vi "BCU诊断标定.vi"(8 "CAN端口":u16(ring), 9 "设备索引号":u16(ring), 10 "CAN卡类型":u32(ring)=21) -> ()   [LabVIEW 2013] (continued)
                  n4261 = call "多帧发送机制(EV05).vi"("can卡类型"=w6108, "设备索引号"=w6107, "CAN端口"=w6106, "命令"=w6105, "板号"=w6102, "命令序号"=w6104, "输入数据"=dbl[] [0.0]) -> ()  [unwired: 1 in, 12 out]
                  n4262 = local write "命令序号"(w6104) -> ()
                }
              }
            }
            frame #1 {
              n4263 = while {
                tunnel: [w6110] -> w6109
                i -> [w6115]
                stop <- w6112 stop-if-true
                n4264 = global read "EV05全局变量1.vi" "写入超时"() -> (w6110:bool)
                n4265 = Greater Or Equal?(x=w6115, y=25) -> (x >= y?=w6113:bool)
                n4266 = Or(x=w6110, y=w6113) -> (x .or. y?=w6112:bool)
                n4267 = Wait Until Next ms Multiple(millisecond multiple=u32 100 ("毫秒倍数")) -> ()  [unwired: 1 out]
              }
            }
            frame #2 {
              n4268 = case shown="假" w6116 {
                frame False {
                  n4269 = control-ref of="结果"() -> (w6118:refnum<vi>)
                  n4270 = Concatenate Strings("项目软件版本" ("字符串"), "     读取失败" ("字符串")) -> (w6121:string)
                  n4271 = Build Array(w6121) -> (w6120:string[])
                  n4272 = call "表格编辑(版本读取).vi"("新元素/子数组"=w6120, "活动单元格:单元格背景色"=u32 16740749, "MCListbox引用句柄"=w6118) -> ()  [unwired: 9 out]
                }
                frame True {
                }
              }
              n4273 = call <vilib>:"Unset Busy.vi"() -> ()  [unwired: 2 in, 10 out]
            }
          }
        }
        frame "读取故障状态" {
          n4274 = stacked-sequence {
            seq-local: [_ w6147 _] -> [_ _ w6154]
            frame #0 {
              n4275 = local read "设备索引号"() -> (w6124:u16)
              n4276 = local read "CAN卡类型"() -> (w6125:u32)
              n4277 = local read "CAN端口"() -> (w6123:u16)
              n4278 = stacked-sequence {
                tunnel: w6125 -> [w6128 w6137]
                tunnel: w6124 -> [w6127 w6136]
                tunnel: w6123 -> [w6126 w6135]
                frame #0 {
                  n4279 = dll-call lib="PTH1mabs FBluewave New EnergySVN_WorkBMS_Monitor_Bnet01trunk参数设置data\nkerneldlls\nusbcan.dll" fn="VCI_ClearBuffer"("DeviceType"=w6128, "DeviceInd"=w6127, "CANInd"=w6126) -> (error out=w6129:errorcluster)  [unwired: 4 in, 4 out]
                  n4280 = call <vilib>:"Clear Errors.vi"("error in (no error)"=w6129) -> ()  [unwired: 6 in, 1 out]
                }
                frame #1 {
                  n4281 = local read "从板板号 2"() -> (w6130:u8)
                  n4282 = case shown="1..30" w6130 {
                    tunnel: [u8 133 ("命令") u8 4 ("命令")] -> w6134
                    frame 0, Default {
                    }
                    frame 1..30 {
                    }
                  }
                  n4283 = local read "状态选择"() -> (w6132:T18)
                  n4284 = local write "命令"(w6134) -> ()
                  n4285 = case shown="\"预充电故障,继电器驱动故障\"" w6132 {
                    tunnel: [1 2 3 4 5 6 7] -> w6131
                    frame "电压,内总电压,外总电压,温度,电流,绝缘,系统时钟,充电均衡,放电均衡", Default {
                    }
                    frame "CPU,CPU内部EE存储器,CPU内部FLASH,内部EE存储器,45db存储器" {
                    }
                    frame "CAN检测故障" {
                    }
                    frame "软件故障" {
                    }
                    frame "RS485,RS232检测故障" {
                    }
                    frame "DI,DO,AI,AO检测故障" {
                    }
                    frame "预充电故障,继电器驱动故障" {
                    }
                  }
                  n4286 = call "多帧发送机制(EV05).vi"("can卡类型"=w6137, "设备索引号"=w6136, "CAN端口"=w6135, "命令"=w6134, "板号"=w6130, "命令序号"=w6131, "输入数据"=dbl[] [0.0]) -> ()  [unwired: 1 in, 12 out]
                  n4287 = local write "命令序号"(w6131) -> ()
                }
              }
            }
            frame #1 {
              n4288 = while {
                tunnel: [w6148] -> w6147
                i -> [w6153]
                stop <- w6150 stop-if-true
                n4289 = global read "EV05全局变量1.vi" "写入超时"() -> (w6148:bool)
                n4290 = Greater Or Equal?(x=w6153, y=25) -> (x >= y?=w6151:bool)
                n4291 = Or(x=w6148, y=w6151) -> (x .or. y?=w6150:bool)
                n4292 = Wait Until Next ms Multiple(millisecond multiple=u32 100 ("毫秒倍数")) -> ()  [unwired: 1 out]
              }
            }
            frame #2 {
              n4293 = case shown="真" w6154 {
                frame False {
                  n4294 = Concatenate Strings("故障信息" ("字符串"), "     读取失败" ("字符串")) -> (w6156:string)
                  n4295 = One Button Dialog(message=w6156, button name ("OK")="确定" ("按钮名称（“确定”）")) -> ()  [unwired: 1 out]
                }
                frame True {
                  n4296 = One Button Dialog(message="故障信息读取完成" ("字符串"), button name ("OK")="确定" ("按钮名称（“确定”）")) -> ()  [unwired: 1 out]
                }
              }
              n4297 = call <vilib>:"Unset Busy.vi"() -> ()  [unwired: 2 in, 10 out]
            }
          }
        }
        frame "平台软件版本读取" {
          n4298 = stacked-sequence {
            seq-local: [_ w6176 _] -> [_ _ w6183]
            frame #0 {
              n4299 = local read "设备索引号"() -> (w6163:u16)
              n4300 = local read "CAN卡类型"() -> (w6164:u32)
              n4301 = local read "CAN端口"() -> (w6162:u16)
              n4302 = stacked-sequence {
                tunnel: w6164 -> [w6167 w6175]
                tunnel: w6163 -> [w6166 w6174]
                tunnel: w6162 -> [w6165 w6173]
                tunnel: u8 137 ("命令") -> [_ w6172]
                frame #0 {
                  n4303 = dll-call lib="PTH1mabs FBluewave New EnergySVN_WorkBMS_Monitor_Bnet01trunk参数设置data\nkerneldlls\nusbcan.dll" fn="VCI_ClearBuffer"("DeviceType"=w6167, "DeviceInd"=w6166, "CANInd"=w6165) -> (error out=w6168:errorcluster)  [unwired: 4 in, 4 out]
                  n4304 = call <vilib>:"Clear Errors.vi"("error in (no error)"=w6168) -> ()  [unwired: 6 in, 1 out]
                }
                frame #1 {
                  w6171 = u32 2 ("命令序号")
                  n4305 = local read "从板板号"() -> (w6169:u8)
                  n4306 = local write "命令"(w6172) -> ()
                  n4307 = call "多帧发送机制(EV05).vi"("can卡类型"=w6175, "设备索引号"=w6174, "CAN端口"=w6173, "命令"=w6172, "板号"=w6169, "命令序号"=w6171, "输入数据"=dbl[] [0.0]) -> ()  [unwired: 1 in, 12 out]
                  n4308 = local write "命令序号"(w6171) -> ()
                }
              }
            }
            frame #1 {
              n4309 = while {
                tunnel: [w6177] -> w6176
                i -> [w6182]
                stop <- w6179 stop-if-true
                n4310 = global read "EV05全局变量1.vi" "写入超时"() -> (w6177:bool)
                n4311 = Greater Or Equal?(x=w6182, y=25) -> (x >= y?=w6180:bool)
                n4312 = Or(x=w6177, y=w6180) -> (x .or. y?=w6179:bool)
                n4313 = Wait Until Next ms Multiple(millisecond multiple=u32 100 ("毫秒倍数")) -> ()  [unwired: 1 out]
              }
            }
            frame #2 {
              n4314 = case shown="假" w6183 {
                frame False {
                  n4315 = control-ref of="结果"() -> (w6186:refnum<vi>)
                  n4316 = Concatenate Strings("平台软件版本" ("字符串"), "     读取失败" ("字符串")) -> (w6188:string)
                  n4317 = Build Array(w6188) -> (w6185:string[])
                  n4318 = call "表格编辑(版本读取).vi"("新元素/子数组"=w6185, "活动单元格:单元格背景色"=u32 16740749, "MCListbox引用句柄"=w6186) -> ()  [unwired: 9 out]
                }
                frame True {
                }
              }
              n4319 = call <vilib>:"Unset Busy.vi"() -> ()  [unwired: 2 in, 10 out]
            }
          }
        }
        frame "模块软件版本读取" {
          n4320 = local read "从板板号"() -> (w6190:u8)
          n4321 = local read "模块软件版本"() -> (w6191:T1)
          n4322 = case shown="\"全部读取\"" w6191 {
            selector: w6191 -> [w6192 w6236]
            tunnel: w6190 -> [_ w6235]
            frame "BCUMCAL", Default {
              n4323 = stacked-sequence {
                seq-local: [_ _ w6218 _] -> [_ _ _ w6225]
                tunnel: w6192 -> [_ w6198 _ w6226]
                frame #0 {
                  w6197 = FALSE ("写?")
                  n4324 = call <vilib>:"Set Busy.vi"("disable click? (T)"=FALSE) -> ()  [unwired: 3 in, 8 out]
                  n4325 = local write "写?"(w6197) -> ()
                  n4326 = global write "EV05全局变量1.vi" "流控帧 2"(TRUE ("流控帧 2")) -> ()
                  n4327 = global write "EV05全局变量1.vi" "写入超时"(w6197) -> ()
                  n4328 = local write "控制1"(TRUE ("控制1")) -> ()
                  n4329 = local write "消除"(TRUE ("消除")) -> ()
                }
                frame #1 {
                  n4330 = Quotient & Remainder(x=w6198, y=256) -> (x-y*floor(x/y)=w6199:i32, floor(x/y)=w6200:i32)
                  n4331 = Build Array(w6200, w6199, u8 0 ("板号")) -> (w6203:i32[])
                  n4332 = local read "设备索引号"() -> (w6205:u16)
                  n4333 = local read "CAN卡类型"() -> (w6206:u32)
                  n4334 = local read "CAN端口"() -> (w6204:u16)
                  n4335 = stacked-sequence {
                    tunnel: w6206 -> [w6209 w6217]
                    tunnel: w6205 -> [w6208 w6216]
                    tunnel: w6204 -> [w6207 w6215]
                    tunnel: w6203 -> [_ w6214]
                    frame #0 {
                      n4336 = dll-call lib="PTH1mabs FBluewave New EnergySVN_WorkBMS_Monitor_Bnet01trunk参数设置data\nkerneldlls\nusbcan.dll" fn="VCI_ClearBuffer"("DeviceType"=w6209, "DeviceInd"=w6208, "CANInd"=w6207) -> (error out=w6210:errorcluster)  [unwired: 4 in, 4 out]
                      n4337 = call <vilib>:"Clear Errors.vi"("error in (no error)"=w6210) -> ()  [unwired: 6 in, 1 out]
                    }
                    frame #1 {
                      w6213 = u8 137 ("命令")
                      w6211 = u32 3 ("命令序号")
                      n4338 = local read "从板板号"() -> (w6212:u8)
                      n4339 = local write "命令"(w6213) -> ()
                      n4340 = call "多帧发送机制(EV05).vi"("can卡类型"=w6217, "设备索引号"=w6216, "CAN端口"=w6215, "命令"=w6213, "板号"=w6212, "命令序号"=w6211, "输入数据"=w6214) -> ()  [unwired: 1 in, 12 out]
                      n4341 = local write "命令序号"(w6211) -> ()
                    }
                  }
                }
                frame #2 {
                  n4342 = while {
                    tunnel: [w6219] -> w6218
                    i -> [w6224]
                    stop <- w6220 stop-if-true
                    n4343 = global read "EV05全局变量1.vi" "写入超时"() -> (w6219:bool)
                    n4344 = Greater Or Equal?(x=w6224, y=25) -> (x >= y?=w6221:bool)
                    n4345 = Or(x=w6219, y=w6221) -> (x .or. y?=w6220:bool)
                    n4346 = Wait Until Next ms Multiple(millisecond multiple=u32 100 ("毫秒倍数")) -> ()  [unwired: 1 out]
                  }
                }
                frame #3 {
                  n4347 = call <vilib>:"Unset Busy.vi"() -> ()  [unwired: 2 in, 10 out]
                  n4348 = case shown="假" w6225 {
                    tunnel: w6226 -> [w6228 _]
                    frame False {
                      n4349 = Number To Decimal String(number=w6228) -> (decimal integer string=w6229:string)  [unwired: 1 out]
                      n4350 = control-ref of="结果"() -> (w6230:refnum<vi>)
                      n4351 = Concatenate Strings("模块" ("字符串"), w6229, "     读取失败" ("字符串")) -> (w6233:string)
                      n4352 = Build Array(w6233) -> (w6232:string[])
                      n4353 = call "表格编辑(版本读取).vi"("新元素/子数组"=w6232, "活动单元格:单元格背景色"=u32 16740749, "MCListbox引用句柄"=w6230) -> ()  [unwired: 9 out]
                    }
                    frame True {
                    }
                  }
                }
              }
            }
            frame "全部读取" {
              n4354 = stacked-sequence {
                seq-local: [w6237 _] -> [_ w6275]
                tunnel: w6236 -> [_ w6277]
                tunnel: w6235 -> [w6238 w6276]
                frame #0 {
                  n4355 = stacked-sequence {
                    tunnel: w6238 -> [_ w6247 _]
                    tunnel: [_ _ w6267] -> w6237
                    frame #0 {
                      w6243 = FALSE ("写?")
                      n4356 = control-ref of="模块软件版本 2"() -> (w6241:refnum<vi>)
                      n4357 = call <vilib>:"Set Busy.vi"("disable click? (T)"=FALSE) -> ()  [unwired: 3 in, 8 out]
                      n4358 = local write "写?"(w6243) -> ()
                      n4359 = property class="MCListbox (严格)"(reference=w6241, "ItemNames"=string[][] []) -> ()  [unwired: 1 in, 2 out]
                      n4360 = global write "EV05全局变量1.vi" "写入超时"(w6243) -> ()
                      n4361 = local write "消除"(TRUE ("消除")) -> ()
                      n4362 = local write "控制1"(TRUE ("控制1")) -> ()
                      n4363 = global write "EV05全局变量1.vi" "流控帧 2"(TRUE ("流控帧 2")) -> ()
                      n4364 = local write "MODEL号"(u8[] [] ("MODEL号")) -> ()
                    }
                    frame #1 {
                      n4365 = local read "设备索引号"() -> (w6249:u16)
                      n4366 = local read "CAN卡类型"() -> (w6250:u32)
                      n4367 = local read "CAN端口"() -> (w6248:u16)
                      n4368 = stacked-sequence {
                        tunnel: w6250 -> [w6253 w6266]
                        tunnel: w6249 -> [w6252 w6265]
                        tunnel: w6248 -> [w6251 w6264]
                        tunnel: w6247 -> [_ w6256]
                        frame #0 {
                          n4369 = dll-call lib="PTH1mabs FBluewave New EnergySVN_WorkBMS_Monitor_Bnet01trunk参数设置data\nkerneldlls\nusbcan.dll" fn="VCI_ClearBuffer"("DeviceType"=w6253, "DeviceInd"=w6252, "CANInd"=w6251) -> (error out=w6254:errorcluster)  [unwired: 4 in, 4 out]
                          n4370 = call <vilib>:"Clear Errors.vi"("error in (no error)"=w6254) -> ()  [unwired: 6 in, 1 out]
                        }
                        frame #1 {
                          w6262 = u8 137 ("命令")
                          w6260 = u32 3 ("命令序号")
                          n4371 = Quotient & Remainder(x=u8 0 ("板号"), y=256) -> (x-y*floor(x/y)=w6257:i32, floor(x/y)=w6258:i32)
                          n4372 = local write "命令"(w6262) -> ()
                          n4373 = Build Array(w6258, w6257, u8 0 ("板号")) -> (w6263:i32[])
                          n4374 = call "多帧发送机制(EV05).vi"("can卡类型"=w6266, "设备索引号"=w6265, "CAN端口"=w6264, "命令"=w6262, "板号"=w6256, "命令序号"=w6260, "输入数据"=w6263) -> ()  [unwired: 1 in, 12 out]
                          n4375 = local write "命令序号"(w6260) -> ()
                        }
                      }
                    }
                    frame #2 {
                      n4376 = while {
                        tunnel: [w6269] -> w6267
                        i -> [w6273]
                        stop <- w6270 stop-if-true
                        n4377 = local read "强制停止版本读取"() -> (w6268:bool)
                        n4378 = global read "EV05全局变量1.vi" "写入超时"() -> (w6269:bool)
                        n4379 = Greater Or Equal?(x=w6273, y=35) -> (x >= y?=w6271:bool)
                        n4380 = Compound Arithmetic op=OR(w6268, w6269, w6271) -> (w6270:bool)
                        n4381 = Wait Until Next ms Multiple(millisecond multiple=u32 100 ("毫秒倍数")) -> ()  [unwired: 1 out]
                      }
                    }
                  }
                }
                frame #1 {
                  n4382 = case shown="真" w6275 {
                    tunnel: w6277 -> [_ w6287]
                    tunnel: w6276 -> [_ w6286]
                    frame False {
                      n4383 = control-ref of="结果"() -> (w6279:refnum<vi>)
                      n4384 = Concatenate Strings("模块编号" ("字符串"), "读取失败" ("字符串")) -> (w6282:string)
                      n4385 = Build Array(w6282) -> (w6281:string[])
                      n4386 = call "表格编辑(版本读取).vi"("新元素/子数组"=w6281, "活动单元格:单元格背景色"=u32 16740749, "MCListbox引用句柄"=w6279) -> ()  [unwired: 9 out]
                      n4387 = call <vilib>:"Unset Busy.vi"() -> ()  [unwired: 11 in, 1 out]
                    }
                    frame True {
                      n4388 = local read "MODEL号"() -> (w6285:u8[])
                      n4389 = Array Size(array=w6285) -> (size(s)=w6284:i32)
                      n4390 = for {
                        tunnel: w6287 -> [_]
                        tunnel: w6286 -> [w6290]
                        tunnel: w6285 -> [w6289] mode=indexing
                        tunnel: w6284 -> [w6288]
                        i -> [w6292]
                        n4391 = Increment(x=w6292) -> (x+1=w6291:i32)
                        n4392 = stacked-sequence {
                          seq-local: [_ _ _ w6319 _ _] -> [_ _ _ _ w6328 _]
                          seq-local: [_ w6298 _ _ _ _] -> [_ _ _ _ w6327 _]
                          tunnel: w6291 -> [_ _ _ _ _ w6339]
                          tunnel: w6289 -> [_ w6298 _ _ _ _]
                          tunnel: w6290 -> [_ w6299 _ _ _ _]
                          tunnel: w6288 -> [_ _ _ _ _ w6337]
                          frame #0 {
                            w6294 = FALSE ("写?")
                            n4393 = call <vilib>:"Set Busy.vi"("disable click? (T)"=FALSE) -> ()  [unwired: 3 in, 8 out]
                            n4394 = local write "写?"(w6294) -> ()
                            n4395 = global write "EV05全局变量1.vi" "写入超时"(w6294) -> ()
                            n4396 = global write "EV05全局变量1.vi" "流控帧 2"(TRUE ("流控帧 2")) -> ()
                            n4397 = local write "控制1"(TRUE ("控制1")) -> ()
                            n4398 = local write "消除"(TRUE ("消除")) -> ()
                          }
                          frame #1 {
                            n4399 = local read "设备索引号"() -> (w6301:u16)
                            n4400 = local read "CAN卡类型"() -> (w6302:u32)
                            n4401 = local read "CAN端口"() -> (w6300:u16)
                            n4402 = stacked-sequence {
                              tunnel: w6302 -> [w6305 w6318]
                              tunnel: w6301 -> [w6304 w6317]
                              tunnel: w6300 -> [w6303 w6316]
                              tunnel: w6299 -> [_ w6308]
                              tunnel: w6298 -> [_ w6307]
                              frame #0 {
                                n4403 = dll-call lib="PTH1mabs FBluewave New EnergySVN_WorkBMS_Monitor_Bnet01trunk参数设置data\nkerneldlls\nusbcan.dll" fn="VCI_ClearBuffer"("DeviceType"=w6305, "DeviceInd"=w6304, "CANInd"=w6303) -> (error out=w6306:errorcluster)  [unwired: 4 in, 4 out]
                                n4404 = call <vilib>:"Clear Errors.vi"("error in (no error)"=w6306) -> ()  [unwired: 6 in, 1 out]
                              }
                              frame #1 {
                                w6314 = u8 137 ("命令")
                                w6312 = u32 3 ("命令序号")
                                n4405 = Quotient & Remainder(x=w6307, y=256) -> (x-y*floor(x/y)=w6309:i32, floor(x/y)=w6310:i32)
                                n4406 = local write "命令"(w6314) -> ()
                                n4407 = Build Array(w6310, w6309, u8 0 ("板号")) -> (w6315:i32[])
                                n4408 = call "多帧发送机制(EV05).vi"("can卡类型"=w6318, "设备索引号"=w6317, "CAN端口"=w6316, "命令"=w6314, "板号"=w6308, "命令序号"=w6312, "输入数据"=w6315) -> ()  [unwired: 1 in, 12 out]
                                n4409 = local write "命令序号"(w6312) -> ()
                              }
                            }
                          }
                          frame #2 {
                          }
                          frame #3 {
                            n4410 = while {
                              tunnel: [w6321] -> w6319
                              i -> [w6325]
                              stop <- w6322 stop-if-true
                              n4411 = local read "强制停止版本读取"() -> (w6320:bool)
                              n4412 = global read "EV05全局变量1.vi" "写入超时"() -> (w6321:bool)
                              n4413 = Greater Or Equal?(x=w6325, y=25) -> (x >= y?=w6323:bool)
                              n4414 = Compound Arithmetic op=OR(w6320, w6321, w6323) -> (w6322:bool)
                              n4415 = Wait Until Next ms Multiple(millisecond multiple=u32 100 ("毫秒倍数")) -> ()  [unwired: 1 out]
                            }
                          }
                          frame #4 {
                            n4416 = call <vilib>:"Unset Busy.vi"() -> ()  [unwired: 11 in, 1 out]
                            n4417 = case shown="假" w6328 {
                              tunnel: w6327 -> [w6330 _]
                              frame False {
                                n4418 = control-ref of="结果"() -> (w6332:refnum<vi>)
                                n4419 = Number To Decimal String(number=w6330) -> (decimal integer string=w6331:string)  [unwired: 1 out]
                                n4420 = Concatenate Strings("模块" ("字符串"), w6331, "     读取失败" ("字符串")) -> (w6335:string)
                                n4421 = Build Array(w6335) -> (w6334:string[])
                                n4422 = call "表格编辑(版本读取).vi"("新元素/子数组"=w6334, "活动单元格:单元格背景色"=u32 16740749, "MCListbox引用句柄"=w6332) -> ()  [unwired: 9 out]
                              }
                              frame True {
                              }
                            }
                          }
                          frame #5 {
                            n4423 = Equal?(x=w6337, y=w6339) -> (x = y?=w6338:bool)
                            n4424 = case shown="真" w6338 {
                              frame False {
                              }
                              frame True {
                                n4425 = control-ref of="模块软件版本 2"() -> (w6350:refnum<vi>)
                                n4426 = local read "模块版本名称"() -> (w6349:string[][])
                                n4427 = local read "模块版本值"() -> (w6345:string[][])
                                n4428 = control-ref of="结果"() -> (w6357:refnum<vi>)
                                n4429 = property class="MCListbox (严格)"(reference=w6350) -> ("ItemNames"=w6353:string[][])  [unwired: 1 in, 2 out]
                                n4430 = local read "从板板号"() -> (w6340:u8)
                                n4431 = Concatenate Strings("模块版本读取完成" ("字符串")) -> (w6360:string)
                                n4432 = Build Array(w6360) -> (w6359:string[])
                                n4433 = call "表格编辑(版本读取).vi"("新元素/子数组"=w6359, "活动单元格:单元格背景色"=u32 21937, "MCListbox引用句柄"=w6357) -> ()  [unwired: 9 out]
                                n4434 = Transpose 2D Array(2D array=w6353) -> (transposed array=w6354:string[][])
                                n4435 = local write "强制停止版本读取"(FALSE ("强制停止 2")) -> ()
                                n4436 = local read "模块个数"() -> (w6343:u8[])
                                n4437 = Index Array(array=w6354, index (row) #1=0 ("索引 (行)"), index (row) #2=1 ("索引 (行)")) -> (element #1=w6344:string[], element #2=w6346:string[])  [unwired: 2 in]
                                n4438 = Replace Array Subset(array=w6349, new element=w6344, index (row)=w6340) -> (w6348:string[][])  [unwired: 1 in]
                                n4439 = Replace Array Subset(array=w6345, new element=w6346, index (row)=w6340) -> (w6347:string[][])  [unwired: 1 in]
                                n4440 = local write "模块版本名称"(w6348) -> ()
                                n4441 = local write "模块版本值"(w6347) -> ()
                                n4442 = Array Size(array=w6344) -> (size(s)=w6341:i32)
                                n4443 = Replace Array Subset(array=w6343, new element=w6341, index=w6340) -> (w6342:u8[])
                                n4444 = local write "模块个数"(w6342) -> ()
                              }
                            }
                          }
                        }
                      }
                    }
                  }
                }
              }
            }
          }
        }
        frame "硬件版本读取" {
          n4445 = stacked-sequence {
            seq-local: [_ _ w6368 _] -> [_ _ _ w6375]
            frame #0 {
              w6364 = u8 137 ("命令")
              w6363 = u32 4 ("命令序号")
              n4446 = local read "设备索引号"() -> (w6366:u16)
              n4447 = local read "CAN卡类型"() -> (w6367:u32)
              n4448 = local read "CAN端口"() -> (w6365:u16)
              n4449 = local read "从板板号"() -> (w6361:u8)
              n4450 = local write "命令"(w6364) -> ()
              n4451 = call "多帧发送机制(EV05).vi"("can卡类型"=w6367, "设备索引号"=w6366, "CAN端口"=w6365, "命令"=w6364, "板号"=w6361, "命令序号"=w6363, "输入数据"=dbl[] [0.0]) -> ()  [unwired: 1 in, 12 out]
              n4452 = local write "命令序号"(w6363) -> ()
            }
            frame #1 {
            }
            frame #2 {
              n4453 = while {
                tunnel: [w6369] -> w6368
                i -> [w6374]
                stop <- w6370 stop-if-true
                n4454 = global read "EV05全局变量1.vi" "写入超时"() -> (w6369:bool)
                n4455 = Greater Or Equal?(x=w6374, y=25) -> (x >= y?=w6371:bool)
                n4456 = Or(x=w6369, y=w6371) -> (x .or. y?=w6370:bool)
                n4457 = Wait Until Next ms Multiple(millisecond multiple=u32 100 ("毫秒倍数")) -> ()  [unwired: 1 out]
              }
            }
            frame #3 {
              n4458 = case shown="假" w6375 {
                frame False {
                  n4459 = control-ref of="结果"() -> (w6377:refnum<vi>)
                  n4460 = Concatenate Strings("硬件版本" ("字符串"), "     读取失败" ("字符串")) -> (w6380:string)
                  n4461 = Build Array(w6380) -> (w6379:string[])
                  n4462 = call "表格编辑(版本读取).vi"("新元素/子数组"=w6379, "活动单元格:单元格背景色"=u32 16740749, "MCListbox引用句柄"=w6377) -> ()  [unwired: 9 out]
                }
                frame True {
                }
              }
              n4463 = call <vilib>:"Unset Busy.vi"() -> ()  [unwired: 2 in, 10 out]
            }
          }
        }
        frame "写配置文件" {
          n4464 = disable-structure shown="启用" {
            frame Enabled {
              n4465 = local read "主从选择"() -> (w6388:enum32{"主板", "从板"})
              n4466 = case shown="\"从板\"" w6388 {
                tunnel: [w6407 w6598] -> w6391
                tunnel: ["M0" w6604] -> w6389
                frame "主板", Default {
                  n4467 = stacked-sequence {
                    seq-local: [w6421 _ _ _ _ _ _] -> [_ w6450 _ _ _ _ _]
                    seq-local: [string[] ["电池额定容量", "电池实际容量", "SOC", "SOH", "车牌号", "配置文件版本", "产品编号", "系统时钟"] _ _ _ _ _ _] -> [_ w6445 _ _ _ _ _]
                    seq-local: [_ _ _ _ string[] ["风机开启温度", "风机关闭温度", "加热开启温度", "加热关闭温度", "风机开启温差", "风机关闭温差", "加热关闭温差"] _ _] -> [_ _ _ _ _ w6550 _]
                    seq-local: [_ _ _ _ w6531 _ _] -> [_ _ _ _ _ w6548 _]
                    tunnel: [w6422 _ _ _ _ _ _] -> w6409
                    tunnel: [_ w6452 _ _ _ _ _] -> w6406
                    tunnel: [_ _ w6476 _ _ _ _] -> w6405
                    tunnel: [_ _ _ w6503 _ _ _] -> w6404
                    tunnel: [_ _ _ _ _ w6551 _] -> w6403
                    tunnel: [_ _ _ _ _ _ w6568] -> w6402
                    frame #0 {
                      w6413 = string[] ["", "", "", "", "", "", "", "", "", "", "  "]
                      n4468 = control-ref of="项目信息"() -> (w6441:refnum<vi>)
                      n4469 = property class="Tbl (严格)"(reference=w6441) -> ("Value"=w6417:string[][])  [unwired: 1 in, 2 out]
                      n4470 = control-ref of="项目信息2"() -> (w6435:refnum<vi>)
                      n4471 = Index Array(array=w6417, index (col)=0 ("禁用的索引 (列)")) -> (element=w6418:string[])  [unwired: 1 in]
                      n4472 = property class="Clust (严格)"(reference=w6435) -> ("Value"=w6434:T9)  [unwired: 1 in, 2 out]
                      n4473 = Index Array(array=w6417, index (col)=1 ("禁用的索引 (列)")) -> (element=w6416:string[])  [unwired: 1 in]
                      n4474 = local read "从板个数"() -> (w6440:dbl)
                      n4475 = Number To Decimal String(number=w6440) -> (decimal integer string=w6439:string)  [unwired: 1 out]
                      n4476 = Insert Into Array(array=w6418, new element=w6413) -> (w6415:string[])  [unwired: 1 in]
                      n4477 = Insert Into Array(array=w6416, new element=w6413) -> (w6414:string[])  [unwired: 1 in]
                      n4478 = Unbundle(w6434) -> ("电池额定容量(A)"=w6433:dbl, "电池实际容量(A)"=w6432:dbl, "车架(牌)号"=w6430:string, "配置文件版本"=w6429:string, "SOH(%)"=w6424:dbl, "SOC(%)"=w6423:dbl, "产品编号"=w6428:string, "系统时钟"=w6427:string)  [unwired: 1 out]
                      n4479 = Build Array("从板个数" ("元素"), w6439) -> (w6436:string[])
                      n4480 = Build Array(w6415, w6414) -> (w6411:string[][])
                      n4481 = Transpose 2D Array(2D array=w6411) -> (transposed array=w6410:string[][])
                      n4482 = Build Array(w6433, w6432, w6423, w6424) -> (w6431:dbl[])
                      n4483 = Build Array(w6430, w6429, w6428, w6427) -> (w6425:string[])
                      n4484 = for {
                        tunnel: w6431 -> [w6443] mode=indexing
                        tunnel: [w6442] -> w6426 mode=indexing
                        n4485 = Format Into String(format string="%#f" ("格式字符串"), w6443) -> (resulting string=w6442:string)  [unwired: 2 in, 1 out]
                      }
                      n4486 = Insert Into Array(array=w6410, index (row)=0 ("索引 (行)"), new element=w6436) -> (w6422:string[][])  [unwired: 1 in]
                      n4487 = Insert Into Array(array=w6426, new element=w6425) -> (w6421:string[])  [unwired: 1 in]
                    }
                    frame #1 {
                      n4488 = control-ref of="一级故障"() -> (w6472:refnum<vi>)
                      n4489 = property class="Clust (严格)"(reference=w6472) -> ("Value"=w6471:T10)  [unwired: 1 in, 2 out]
                      n4490 = Unbundle(w6471) -> ("总电压过高"=w6470:dbl, "整组电压不均衡"=w6465:dbl, "SOC过高"=w6458:dbl, "单体电压过高"=w6461:dbl, "总电压过低"=w6469:dbl, "温度过高"=w6468:dbl, "温度过低"=w6467:dbl, "单组电压不均衡"=w6466:dbl, "整组温度不均衡"=w6463:dbl, "单组温度不均衡"=w6464:dbl, "单体电压过低"=w6462:dbl, "充电电流过高"=w6460:dbl, "放电电流过高"=w6459:dbl, "SOC过低"=w6457:dbl, "内阻过大"=w6456:dbl, "极柱温度过高"=w6455:dbl, "SOH过低"=w6454:dbl)
                      n4491 = Build Array(w6470, w6469, w6468, w6467, w6466, w6465, w6464, w6463, w6461, w6462, w6460, w6459, w6458, w6457, w6456, w6455, w6454) -> (w6453:dbl[])
                      n4492 = for {
                        tunnel: w6453 -> [w6474] mode=indexing
                        tunnel: [w6473] -> w6449 mode=indexing
                        n4493 = Format Into String(format string="%#f" ("格式字符串"), w6474) -> (resulting string=w6473:string)  [unwired: 2 in, 1 out]
                      }
                      n4494 = Insert Into Array(array=w6450, new element=w6449) -> (w6448:string[])  [unwired: 1 in]
                      n4495 = Insert Into Array(array=w6445, new element=string[] ["总电压过高一级", "总电压过低一级", "温度过高一级", "温度过低一级", "单组电压不均衡一级", "整组电压不均衡一级", "单组温度不均衡一级", "整组温度不均衡一级", "单体电压过高一级", "单体电压过低一级", "充电电流过高一级", "放电电流过高一级", "SOC过高一级", "SOC过低一级", "内阻过大一级", "极柱温度过高一级", "SOH过低一级"]) -> (w6447:string[])  [unwired: 1 in]
                      n4496 = Build Array(w6447, w6448) -> (w6446:string[][])
                      n4497 = Transpose 2D Array(2D array=w6446) -> (transposed array=w6452:string[][])
                    }
                    frame #2 {
                      n4498 = control-ref of="一级故障 2"() -> (w6477:refnum<vi>)
                      n4499 = property class="Clust (严格)"(reference=w6477) -> ("Value"=w6499:T10)  [unwired: 1 in, 2 out]
                      n4500 = Unbundle(w6499) -> ("总电压过高"=w6498:dbl, "整组电压不均衡"=w6493:dbl, "SOC过高"=w6486:dbl, "单体电压过高"=w6489:dbl, "总电压过低"=w6497:dbl, "温度过高"=w6496:dbl, "温度过低"=w6495:dbl, "单组电压不均衡"=w6494:dbl, "整组温度不均衡"=w6491:dbl, "单组温度不均衡"=w6492:dbl, "单体电压过低"=w6490:dbl, "充电电流过高"=w6488:dbl, "放电电流过高"=w6487:dbl, "SOC过低"=w6485:dbl, "内阻过大"=w6484:dbl, "极柱温度过高"=w6483:dbl, "SOH过低"=w6482:dbl)
                      n4501 = Build Array(w6498, w6497, w6496, w6495, w6494, w6493, w6492, w6491, w6489, w6490, w6488, w6487, w6486, w6485, w6484, w6483, w6482) -> (w6481:dbl[])
                      n4502 = for {
                        tunnel: w6481 -> [w6501] mode=indexing
                        tunnel: [w6500] -> w6480 mode=indexing
                        n4503 = Format Into String(format string="%#f" ("格式字符串"), w6501) -> (resulting string=w6500:string)  [unwired: 2 in, 1 out]
                      }
                      n4504 = Build Array(string[] ["总电压过高二级", "总电压过低二级", "温度过高二级", "温度过低二级", "单组电压不均衡二级", "整组电压不均衡二级", "单组温度不均衡二级", "整组温度不均衡二级", "单体电压过高二级", "单体电压过低二级", "充电电流过高二级", "放电电流过高二级", "SOC过高二级", "SOC过低二级", "内阻过大二级", "极柱温度过高二级", "SOH过低二级"], w6480) -> (w6478:string[][])
                      n4505 = Transpose 2D Array(2D array=w6478) -> (transposed array=w6476:string[][])
                    }
                    frame #3 {
                      n4506 = control-ref of="一级故障 3"() -> (w6504:refnum<vi>)
                      n4507 = property class="Clust (严格)"(reference=w6504) -> ("Value"=w6526:T10)  [unwired: 1 in, 2 out]
                      n4508 = Unbundle(w6526) -> ("总电压过高"=w6525:dbl, "整组电压不均衡"=w6520:dbl, "SOC过高"=w6513:dbl, "单体电压过高"=w6516:dbl, "总电压过低"=w6524:dbl, "温度过高"=w6523:dbl, "温度过低"=w6522:dbl, "单组电压不均衡"=w6521:dbl, "整组温度不均衡"=w6518:dbl, "单组温度不均衡"=w6519:dbl, "单体电压过低"=w6517:dbl, "充电电流过高"=w6515:dbl, "放电电流过高"=w6514:dbl, "SOC过低"=w6512:dbl, "内阻过大"=w6511:dbl, "极柱温度过高"=w6510:dbl, "SOH过低"=w6509:dbl)
                      n4509 = Build Array(w6525, w6524, w6523, w6522, w6521, w6520, w6519, w6518, w6516, w6517, w6515, w6514, w6513, w6512, w6511, w6510, w6509) -> (w6508:dbl[])
                      n4510 = for {
                        tunnel: w6508 -> [w6528] mode=indexing
                        tunnel: [w6527] -> w6507 mode=indexing
                        n4511 = Format Into String(format string="%#f" ("格式字符串"), w6528) -> (resulting string=w6527:string)  [unwired: 2 in, 1 out]
                      }
                      n4512 = Build Array(string[] ["总电压过高三级", "总电压过低三级", "温度过高三级", "温度过低三级", "单组电压不均衡三级", "整组电压不均衡三级", "单组温度不均衡三级", "整组温度不均衡三级", "单体电压过高三级", "单体电压过低三级", "充电电流过高三级", "放电电流过高三级", "SOC过高三级", "SOC过低三级", "内阻过大三级", "极柱温度过高三级", "SOH过低三级"], w6507) -> (w6505:string[][])
                      n4513 = Transpose 2D Array(2D array=w6505) -> (transposed array=w6503:string[][])
                    }
                    frame #4 {
                      n4514 = control-ref of="加热控制参数"() -> (w6541:refnum<vi>)
                      n4515 = property class="Clust (严格)"(reference=w6541) -> ("Value"=w6540:T11)  [unwired: 1 in, 2 out]
                      n4516 = Unbundle(w6540) -> ("风机开启温度"=w6539:dbl, "风机关闭温度"=w6538:dbl, "加热开启温度"=w6537:dbl, "加热关闭温度"=w6536:dbl, "风机开启温差"=w6535:dbl, "风机关闭温差"=w6534:dbl, "加热关闭温差"=w6530:dbl)
                      n4517 = Build Array(w6539, w6538, w6537, w6536, w6535, w6534, w6530) -> (w6533:dbl[])
                      n4518 = for {
                        tunnel: w6533 -> [w6543] mode=indexing
                        tunnel: [w6542] -> w6531 mode=indexing
                        n4519 = Format Into String(format string="%#f" ("格式字符串"), w6543) -> (resulting string=w6542:string)  [unwired: 2 in, 1 out]
                      }
                    }
                    frame #5 {
                      n4520 = control-ref of="充电控制参数"() -> (w6561:refnum<vi>)
                      n4521 = property class="Clust (严格)"(reference=w6561) -> ("Value"=w6563:T12)  [unwired: 1 in, 2 out]
                      n4522 = Unbundle(w6563) -> ("最大允许单体电压"=w6560:dbl, "最大允许总电压"=w6559:dbl, "最小允许单体电压"=w6558:dbl, "最大允许充电电流"=w6557:dbl, "最小允许充电电流"=w6556:dbl, "最大允许充电温度"=w6555:dbl, "最小允许充电温度"=w6554:dbl, "电流步长"=w6553:dbl)
                      n4523 = Build Array(w6560, w6559, w6558, w6557, w6556, w6555, w6554, w6553) -> (w6562:dbl[])
                      n4524 = for {
                        tunnel: w6562 -> [w6565] mode=indexing
                        tunnel: [w6564] -> w6547 mode=indexing
                        n4525 = Format Into String(format string="%#f" ("格式字符串"), w6565) -> (resulting string=w6564:string)  [unwired: 2 in, 1 out]
                      }
                      n4526 = Insert Into Array(array=w6548, new element=w6547) -> (w6546:string[])  [unwired: 1 in]
                      n4527 = Insert Into Array(array=w6550, new element=string[] ["最大允许单体电压", "最大允许总电压", "最小允许单体电压", "最大允许充电电流", "最小允许充电电流", "最大允许充电温度", "最小允许充电温度", "电流步长"]) -> (w6545:string[])  [unwired: 1 in]
                      n4528 = Build Array(w6545, w6546) -> (w6552:string[][])
                      n4529 = Transpose 2D Array(2D array=w6552) -> (transposed array=w6551:string[][])
                    }
                    frame #6 {
                      n4530 = control-ref of="电池信息"() -> (w6589:refnum<vi>)
                      n4531 = property class="Clust (严格)"(reference=w6589) -> ("Value"=w6592:T13)  [unwired: 1 in, 2 out]
                      n4532 = Unbundle(w6592) -> ("电池串联"=w6588:dbl, "电池并联"=w6587:dbl, "累计放电总安时"=w6585:dbl, "电池包额定容量"=w6584:dbl, "电池包额定能量(kWh)"=w6583:dbl, "电池包额定总电压"=w6582:dbl, "累计充电总安时"=w6586:dbl, "电池充满次数"=w6581:dbl, "电池放空次数"=w6580:dbl, "电池充电次数"=w6579:dbl, "电池生产日期"=w6577:string, "电池厂家"=w6576:string, "电池类型"=w6575:string, "电池包组号"=w6574:string, "电池包产权标识"=w6573:string, "电池应用车型"=w6572:string, "实际容量"=w6567:dbl)
                      n4533 = Build Array(w6577, w6576, w6575, w6574, w6573, w6572) -> (w6571:string[])
                      n4534 = Build Array(w6588, w6587, w6586, w6585, w6584, w6583, w6582, w6581, w6580, w6579, w6567) -> (w6578:dbl[])
                      n4535 = for {
                        tunnel: w6578 -> [w6594] mode=indexing
                        tunnel: [w6593] -> w6570 mode=indexing
                        n4536 = Format Into String(format string="%#f" ("格式字符串"), w6594) -> (resulting string=w6593:string)  [unwired: 2 in, 1 out]
                      }
                      n4537 = Insert Into Array(array=w6571, new element=w6570) -> (w6569:string[])  [unwired: 1 in]
                      n4538 = call <vilib>:"Unset Busy.vi"() -> ()  [unwired: 2 in, 10 out]
                      n4539 = Build Array(string[] ["电池生产日期", "电池厂商", "电池类型", "电池包组号", "电池包产权标识", "电池包应用车型", "电池串联", "电池并联", "累计充电总安时", "累计放电总安时", "电池包额定容量", "电池包额定能量", "电池包额定总电压", "电池充满次数", "电池放空次数", "电池充电次数", "实际容量"], w6569) -> (w6590:string[][])
                      n4540 = Transpose 2D Array(2D array=w6590) -> (transposed array=w6568:string[][])
                    }
                  }
                  n4541 = Insert Into Array(array=w6409, index (col)=2 ("禁用的索引 (列)"), new element #1=w6406, new element #2=w6405, new element #3=w6404, new element #4=w6403, new element #5=w6402) -> (w6407:string[][])  [unwired: 1 in]
                }
                frame "从板" {
                  n4542 = local read "从板号"() -> (w6606:u8)
                  n4543 = Number To Decimal String(number=w6606) -> (decimal integer string=w6603:string)  [unwired: 1 out]
                  n4544 = Concatenate Strings("S", w6603) -> (w6604:string)
                  n4545 = Build Array("从板号" ("元素"), w6603) -> (w6601:string[])
                  n4546 = stacked-sequence {
                    seq-local: [string[] ["风机开启温度", "风机关闭温度", "加热开启温度", "加热关闭温度", "风机开启温差", "风机关闭温差", "加热关闭温差"] _ _ _ _ _] -> [_ _ _ w6675 _ _]
                    seq-local: [w6618 _ _ _ _ _] -> [_ _ _ w6671 _ _]
                    seq-local: [_ string[] ["电压过高一级", "电压过低一级", "温度过高一级", "温度过低一级", "电压不均衡一级", "温度不均衡一级", "SOC过低一级"] _ _ _ _] -> [_ _ _ w6674 _ _]
                    seq-local: [_ w6636 _ _ _ _] -> [_ _ _ w6670 _ _]
                    seq-local: [_ _ string[] ["电压过高二级", "电压过低二级", "温度过高二级", "温度过低二级", "电压不均衡二级", "温度不均衡二级", "SOC过低二级"] _ _ _] -> [_ _ _ w6673 _ _]
                    seq-local: [_ _ w6651 _ _ _] -> [_ _ _ w6669 _ _]
                    tunnel: w6601 -> [w6631 _ _ _ _ _]
                    tunnel: [w6620 _ _ _ _ _] -> w6599
                    tunnel: [_ _ _ w6676 _ _] -> w6597
                    tunnel: [_ _ _ _ w6714 _] -> w6596
                    tunnel: [_ _ _ _ _ w6750] -> _
                    frame #0 {
                      w6611 = string[] ["", "", "", "", "", "", "", "", "", "", "  "]
                      n4547 = control-ref of="项目信息 2"() -> (w6630:refnum<vi>)
                      n4548 = property class="Tbl (严格)"(reference=w6630) -> ("Value"=w6608:string[][])  [unwired: 1 in, 2 out]
                      n4549 = control-ref of="加热控制参数"() -> (w6622:refnum<vi>)
                      n4550 = property class="Clust (严格)"(reference=w6622) -> ("Value"=w6629:T11)  [unwired: 1 in, 2 out]
                      n4551 = Unbundle(w6629) -> ("风机开启温度"=w6628:dbl, "风机关闭温度"=w6627:dbl, "加热开启温度"=w6626:dbl, "加热关闭温度"=w6625:dbl, "风机开启温差"=w6624:dbl, "风机关闭温差"=w6623:dbl, "加热关闭温差"=w6617:dbl)
                      n4552 = Build Array(w6628, w6627, w6626, w6625, w6624, w6623, w6617) -> (w6621:dbl[])
                      n4553 = for {
                        tunnel: w6621 -> [w6634] mode=indexing
                        tunnel: [w6633] -> w6618 mode=indexing
                        n4554 = Format Into String(format string="%#f" ("格式字符串"), w6634) -> (resulting string=w6633:string)  [unwired: 2 in, 1 out]
                      }
                      n4555 = Index Array(array=w6608, index (col)=0 ("禁用的索引 (列)")) -> (element=w6615:string[])  [unwired: 1 in]
                      n4556 = Index Array(array=w6608, index (col)=1 ("禁用的索引 (列)")) -> (element=w6614:string[])  [unwired: 1 in]
                      n4557 = Insert Into Array(array=w6615, new element=w6611) -> (w6613:string[])  [unwired: 1 in]
                      n4558 = Insert Into Array(array=w6614, new element=w6611) -> (w6612:string[])  [unwired: 1 in]
                      n4559 = Build Array(w6613, w6612) -> (w6609:string[][])
                      n4560 = Transpose 2D Array(2D array=w6609) -> (transposed array=w6607:string[][])
                      n4561 = Insert Into Array(array=w6607, index (row)=0 ("索引 (行)"), new element=w6631) -> (w6620:string[][])  [unwired: 1 in]
                    }
                    frame #1 {
                      n4562 = control-ref of="一级故障(从板)"() -> (w6647:refnum<vi>)
                      n4563 = property class="Clust (严格)"(reference=w6647) -> ("Value"=w6646:T15)  [unwired: 1 in, 2 out]
                      n4564 = Unbundle(w6646) -> ("电压过高"=w6645:dbl, "电压过低"=w6644:dbl, "温度过高"=w6643:dbl, "温度过低"=w6642:dbl, "电压不均衡(V)"=w6641:dbl, "温度不均衡"=w6640:dbl, "SOC过低"=w6639:dbl)
                      n4565 = Build Array(w6645, w6644, w6643, w6642, w6641, w6640, w6639) -> (w6638:dbl[])
                      n4566 = for {
                        tunnel: w6638 -> [w6649] mode=indexing
                        tunnel: [w6648] -> w6636 mode=indexing
                        n4567 = Format Into String(format string="%#f" ("格式字符串"), w6649) -> (resulting string=w6648:string)  [unwired: 2 in, 1 out]
                      }
                    }
                    frame #2 {
                      n4568 = control-ref of="二级故障(从板)"() -> (w6653:refnum<vi>)
                      n4569 = property class="Clust (严格)"(reference=w6653) -> ("Value"=w6662:T15)  [unwired: 1 in, 2 out]
                      n4570 = Unbundle(w6662) -> ("电压过高"=w6661:dbl, "电压过低"=w6660:dbl, "温度过高"=w6659:dbl, "温度过低"=w6658:dbl, "电压不均衡(V)"=w6657:dbl, "温度不均衡"=w6656:dbl, "SOC过低"=w6655:dbl)
                      n4571 = Build Array(w6661, w6660, w6659, w6658, w6657, w6656, w6655) -> (w6654:dbl[])
                      n4572 = for {
                        tunnel: w6654 -> [w6664] mode=indexing
                        tunnel: [w6663] -> w6651 mode=indexing
                        n4573 = Format Into String(format string="%#f" ("格式字符串"), w6664) -> (resulting string=w6663:string)  [unwired: 2 in, 1 out]
                      }
                    }
                    frame #3 {
                      n4574 = control-ref of="三级故障(从板)"() -> (w6677:refnum<vi>)
                      n4575 = property class="Clust (严格)"(reference=w6677) -> ("Value"=w6687:T15)  [unwired: 1 in, 2 out]
                      n4576 = Unbundle(w6687) -> ("电压过高"=w6686:dbl, "电压过低"=w6685:dbl, "温度过高"=w6684:dbl, "温度过低"=w6683:dbl, "电压不均衡(V)"=w6682:dbl, "温度不均衡"=w6681:dbl, "SOC过低"=w6680:dbl)
                      n4577 = Build Array(w6686, w6685, w6684, w6683, w6682, w6681, w6680) -> (w6679:dbl[])
                      n4578 = for {
                        tunnel: w6679 -> [w6689] mode=indexing
                        tunnel: [w6688] -> w6668 mode=indexing
                        n4579 = Format Into String(format string="%#f" ("格式字符串"), w6689) -> (resulting string=w6688:string)  [unwired: 2 in, 1 out]
                      }
                      n4580 = Insert Into Array(array=w6675, new element #1=w6674, new element #2=w6673, new element #3=string[] ["电压过高三级", "电压过低三级", "温度过高三级", "温度过低三级", "电压不均衡三级", "温度不均衡三级", "SOC过低三级"]) -> (w6666:string[])  [unwired: 1 in]
                      n4581 = Insert Into Array(array=w6671, new element #1=w6670, new element #2=w6669, new element #3=w6668) -> (w6667:string[])  [unwired: 1 in]
                      n4582 = Build Array(w6666, w6667) -> (w6678:string[][])
                      n4583 = Transpose 2D Array(2D array=w6678) -> (transposed array=w6676:string[][])
                    }
                    frame #4 {
                      n4584 = control-ref of="快换(从板)"() -> (w6713:refnum<vi>)
                      n4585 = property class="Clust (严格)"(reference=w6713) -> ("Value"=w6726:T16)  [unwired: 1 in, 2 out]
                      n4586 = Unbundle(w6726) -> ("串联数"=w6725:dbl, "并联数"=w6724:dbl, "电池厂家"=w6723:dbl, "电池类型"=w6722:dbl, "额定能量"=w6721:dbl, "额定容量"=w6720:dbl, "实际容量"=w6719:dbl, "额定总压"=w6712:dbl, "产权标识"=w6711:dbl, "应用车型"=w6710:dbl, "电池包组号"=w6709:dbl, "SOC"=w6707:dbl, "充电总安时"=w6706:dbl, "放电总安时"=w6705:dbl, "放空次数"=w6704:dbl, "充满次数"=w6703:dbl, "充电次数"=w6702:dbl, "车牌号"=w6692:string, "生产日期"=w6691:string, "最大允许单体电压"=w6701:dbl, "最大允许总电压"=w6700:dbl, "最大允许温度"=w6699:dbl, "最小允许温度"=w6698:dbl, "最大允许充电电流"=w6697:dbl, "最小允许充电电流"=w6696:dbl, "最小允许单体电压"=w6695:dbl, "电流步长"=w6694:dbl, "电池包序号"=w6693:dbl)
                      n4587 = Build Array(w6725, w6724, w6723, w6722, w6721, w6720, w6719, w6712, w6711, w6710, w6709, w6707, w6706, w6705, w6704, w6703, w6702, w6701, w6700, w6699, w6698, w6697, w6696, w6695, w6694, w6693) -> (w6718:dbl[])
                      n4588 = for {
                        tunnel: w6718 -> [w6728] mode=indexing
                        tunnel: [w6727] -> w6716 mode=indexing
                        n4589 = Format Into String(format string="%#f" ("格式字符串"), w6728) -> (resulting string=w6727:string)  [unwired: 2 in, 1 out]
                      }
                      n4590 = Insert Into Array(array=w6716, new element #1=w6692, new element #2=w6691) -> (w6708:string[])  [unwired: 1 in]
                      n4591 = call <vilib>:"Unset Busy.vi"() -> ()  [unwired: 2 in, 10 out]
                      n4592 = Build Array(string[] ["电池串联数", "电池并联数", "电池厂家", "额定能量", "额定容量", "实际容量", "额定总压", "产权标识", "应用车型", "电池包组号", "SOC", "充电总安时", "放电总安时", "放空次数", "充满次数", "充电次数", "最大允许单体电压", "最大允许总电压", "最大允许温度", "最小允许温度", "最大允许充电电流", "最小允许充电电流", "最小允许单体电压", "电流步长", "电池包序号"], w6708) -> (w6717:string[][])
                      n4593 = Transpose 2D Array(2D array=w6717) -> (transposed array=w6714:string[][])
                    }
                    frame #5 {
                      n4594 = local read "均衡参数"() -> (w6749:T17)
                      n4595 = Unbundle(w6749) -> ("充电结束电压(90%)"=w6741:sgl, "充电结束电压(91%)"=w6740:sgl, "充电结束电压(92%)"=w6739:sgl, "充电结束电压(93%)"=w6738:sgl, "充电结束电压(94%)"=w6737:sgl, "均衡计算-电压高阀值1级"=w6748:sgl, "均衡计算-电压高阀值2级"=w6747:sgl, "均衡计算-电压低阀值1级"=w6746:sgl, "均衡计算-电压低阀值2级"=w6745:sgl, "均衡计算-最低电压阀值"=w6744:sgl, "均衡停止-最低电压阀值"=w6743:sgl, "均衡计算-电压极差阀值"=w6742:sgl, "充电结束电压(95%)"=w6736:sgl, "充电结束电压(96%)"=w6735:sgl, "充电结束电压(97%)"=w6734:sgl, "充电结束电压(98%)"=w6733:sgl, "充电结束电压(99%)"=w6732:sgl, "充电结束电压(100%)"=w6731:sgl)
                      n4596 = Build Array(w6748, w6747, w6746, w6745, w6744, w6743, w6742, w6741, w6740, w6739, w6738, w6737, w6736, w6735, w6734, w6733, w6732, w6731) -> (w6753:sgl[])
                      n4597 = for {
                        tunnel: w6753 -> [w6755] mode=indexing
                        tunnel: [w6754] -> w6730 mode=indexing
                        n4598 = Format Into String(format string="%#f" ("格式字符串"), w6755) -> (resulting string=w6754:string)  [unwired: 2 in, 1 out]
                      }
                      n4599 = call <vilib>:"Unset Busy.vi"() -> ()  [unwired: 2 in, 10 out]
                      n4600 = Build Array(string[] ["均衡计算-电压高阀值1级", "均衡计算-电压高阀值2级", "均衡计算-电压低阀值1级", "均衡计算-电压低阀值2级", "均衡计算-最低电压阀值", "均衡停止-最低电压阀值", "均衡计算-电压极差阀值", "充电结束电压(90%)", "充电结束电压(91%)", "充电结束电压(92%)", "充电结束电压(93%)", "充电结束电压(94%)", "充电结束电压(95%)", "充电结束电压(96%)", "充电结束电压(97%)", "充电结束电压(98%)", "充电结束电压(99%)", "充电结束电压(100%)"], w6730) -> (w6752:string[][])
                      n4601 = Transpose 2D Array(2D array=w6752) -> (transposed array=w6750:string[][])
                    }
                  }
                  n4602 = Insert Into Array(array=w6599, index (col)=2 ("禁用的索引 (列)"), new element #1=w6597, new element #2=w6596) -> (w6598:string[][])  [unwired: 1 in]
                }
              }
              n4603 = call "当前时间解析-8.6.vi"() -> ("名称格式时间"=w6390:string)  [unwired: 1 in, 18 out]
              n4604 = Concatenate Strings(w6390, w6389) -> (w6387:string)
              n4605 = call <vilib>:"Application Directory.vi"() -> ("Application Directory"=w6384:path)
              n4606 = call "文件对话框2"("start path"=w6384, "prompt"="选择保存的路径", "default name"=w6387) -> ("selected path"=w6385:path, "cancelled"=w6383:bool, "error out"=w6382:errorcluster)  [unwired: 9 in, 1 out]
              n4607 = call <vilib>:"Clear Errors.vi"("error in (no error)"=w6382) -> ()  [unwired: 6 in, 1 out]
              n4608 = case shown="假" w6383 {
                tunnel: w6391 -> [w6396 _]
                tunnel: w6385 -> [w6392 _]
                frame False {
                  n4609 = call-poly <vilib>:"Write To Spreadsheet File.vi"("append to file? (new file:F)"=FALSE, "2D data"=w6396, "file path (dialog if empty)"=w6392) -> ("new file path (Not A Path if cancelled)"=w6394:path)  [unwired: 3 in, 2 out]
                  n4610 = Path To String(path=w6394) -> (string=w6393:string)
                  n4611 = stacked-sequence {
                    tunnel: w6393 -> [w6399]
                    frame #0 {
                      n4612 = Concatenate Strings("保存完成,路径为:" ("字符串"), w6399) -> (w6400:string)
                      n4613 = One Button Dialog(message=w6400, button name ("OK")="是" ("按钮名称（“确定”）")) -> ()  [unwired: 1 out]
                    }
                  }
                }
                frame True {
                }
              }
            }
            frame Disabled {
              n4614 = stacked-sequence {
                seq-local: [w6770] -> [_]
                frame #0 {
                  n4615 = local read "项目信息"() -> (w6772:string[][])
                  n4616 = local read "项目信息2"() -> (w6769:T9)
                  n4617 = Array Subset(array=w6772, index (row)=0 ("索引"), index (col)=0 ("索引"), length (col)=2 ("索引")) -> (w6775:string[][])  [unwired: 1 in]
                  n4618 = local read "一级故障"() -> ()  [unwired: 1 out]
                  n4619 = local read "从板个数"() -> (w6770:dbl)
                  n4620 = Unbundle(w6769) -> ("电池额定容量(A)"=w6768:dbl, "电池实际容量(A)"=w6767:dbl, "车架(牌)号"=w6761:string, "配置文件版本"=w6760:string, "SOH(%)"=w6765:dbl, "SOC(%)"=w6766:dbl, "产品编号"=w6762:string)  [unwired: 2 out]
                  n4621 = Index Array(array=w6775, index (col) #1=1 ("禁用的索引 (列)"), index (col) #2=0 ("索引 (列)")) -> (element #1=w6759:string[], element #2=w6758:string[])  [unwired: 2 in]
                  n4622 = Build Array(w6768, w6767, w6766, w6765) -> (w6764:dbl[])
                  n4623 = Number To Decimal String(number=w6770) -> ()  [unwired: 1 in, 1 out]
                  n4624 = for {
                    tunnel: w6764 -> [w6780] mode=indexing
                    tunnel: [w6779] -> w6763 mode=indexing
                    n4625 = Format Into String(format string="%#f" ("格式字符串"), w6780) -> (resulting string=w6779:string)  [unwired: 2 in, 1 out]
                  }
                  n4626 = Insert Into Array(array=w6763, new element #1=w6762, new element #2=w6761, new element #3=w6760, new element #4=w6759) -> ()  [unwired: 1 in, 1 out]
                  n4627 = Insert Into Array(array=string[] ["电池额定容量", "电池实际容量", "SOC", "SOH", "产品编号", "车架(牌)号", "配置文件版本"], new element=w6758) -> ()  [unwired: 1 in, 1 out]
                }
              }
            }
          }
        }
        frame "读配置文件" {
        }
      }
    }
    frame Error {
    }
  }
  n4628 = Release Queue(queue=w39, force destroy? (F)=TRUE ("强制销毁？(F)"), error in (no error)=w38) -> (error out=w41:errorcluster)  [unwired: 2 out]
  n4629 = call <vilib>:"Clear Errors.vi"("error in (no error)"=w41) -> ()  [unwired: 7 out]
  n4630 = local write "面板选择"(T7."读写参数" ("面板选择")) -> ()
